vi "ABFL1dll.vi"(8 "error in (no error)":errorcluster, 11 "Inputs":T2) -> (0 "error out":errorcluster, 3 "Outputs":T1)   [LabVIEW 2015]
doc: "SINGLE-PHASE FLASH SUBROUTINES\n\nsubroutine ABFL1dll(a, b, z, kph, ab, dmin, dmax, t, p, D, ierr, herr, ab_length, herr_length)\n\nGeneral single-phase flash routine given two inputs and composition. \n\nValid input properties are temperature, pressure, density, energy, enthalpy, or entropy. \n\nThe character string ab specifies the inputs, which can be: T, P,D, E, H, S. An input of ‘EH’ (or ‘HE’) is not supported. The letters in this string must be uppercase.\n\nCare must be taken when sending inputs of T, P, or D, so that the same variable is not sent twice. For example,\nthe following would be wrong: call ABFL1 (‘TH’,T,H,z,kph,0,0,Dmin,Dmax,T,P,D,ierr,herr) \nRather, the following are examples of correct inputs: call ABFL1 (‘TH’,T,H,z,kph,0,0,Dmin,Dmax,tt,P, D,ierr,herr)\ncall ABFL1 (‘TP’,T,P,z,kph,0,0,Dmin,Dmax,tt,pp,D,ierr,herr) call ABFL1 (‘DS’,D,S,z,kph,0,0,Dmin,Dmax,T, P,dd,ierr,herr)\n\nThis routine accepts only single-phase inputs, it is intended primarily for use with the more general flash routine\nABFLSH, but can be called independently for increased calculation speed if the inputs are know to be singlephase.\nThis will avoid the call to the flash routines to determine the phase of the inputs. If this routine is called,\nbut the inputs are 2-phase, either an incorrect root or a metastable state will be returned (which is OK if the\nmetastable state is desired).\n\nINPUTS:\na -- First property (either temperature, pressure, density, entropy)\nb -- Second property (pressure, density, energy, enthalpy, or entropy)\nz -- Composition (array of mole fractions)\nkph -- Phase flag: 1 - Liquid (kph is only needed for TP inputs) 2 - Vapor\nab -- Character*2 string defining the inputs, e.g., ‘TH’ or ‘PS’ Valid characters\n are: T, P, D, E, H, S\ndmin -- Lower bound on density [mol/L] (for T inputs)\ndmax -- Upper bound on density [mol/L] (for T inputs)\n\nOUTPUTS:\nt -- Temperature [K]\np -- Pressure [kPa]\nD -- Molar density [mol/L]\nierr -- Error flag: 0 Successful, 248 Single-phase iteration did not converge\nherr -- Error string (character*255 variable if ierr<>0)\nab_length -- length of variable ab (default: 2)\nherr_length -- length of variable herr (default: 255) Flags ierr flags"
uses:
  REFPROP.dll
panel:
  # "REFPROP-ABFL1dll.vi"
  # "void  ABFL1dll(double *a, double *b, double *z, int32_t *kph, CStr ab, double *dmin, double *dmax, double *t, double *p, double *D, int32_t *ierr, CStr herr, int32_t ab_length, int32_t herr_length)"
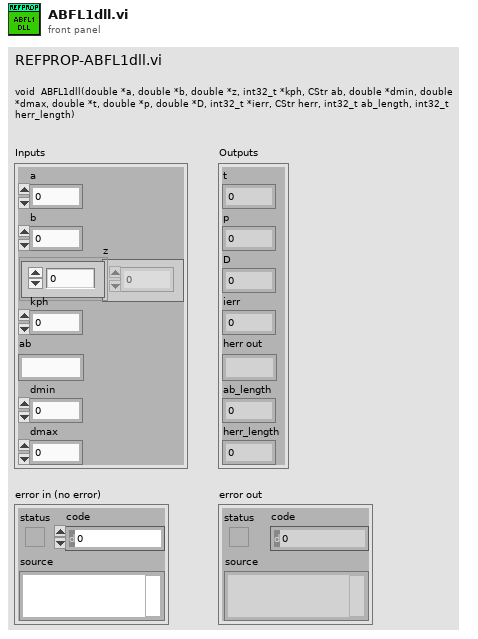
[diagram p1: front panel]
types:
  T1 = cluster{"t":dbl, "p":dbl, "D":dbl, "ierr":i32, "herr out":string, "ab_length":i32, "herr_length":i32}
  T2 = cluster{"a":dbl, "b":dbl, "z":dbl[], "kph":i32, "ab":string, "dmin":dbl, "dmax":dbl}
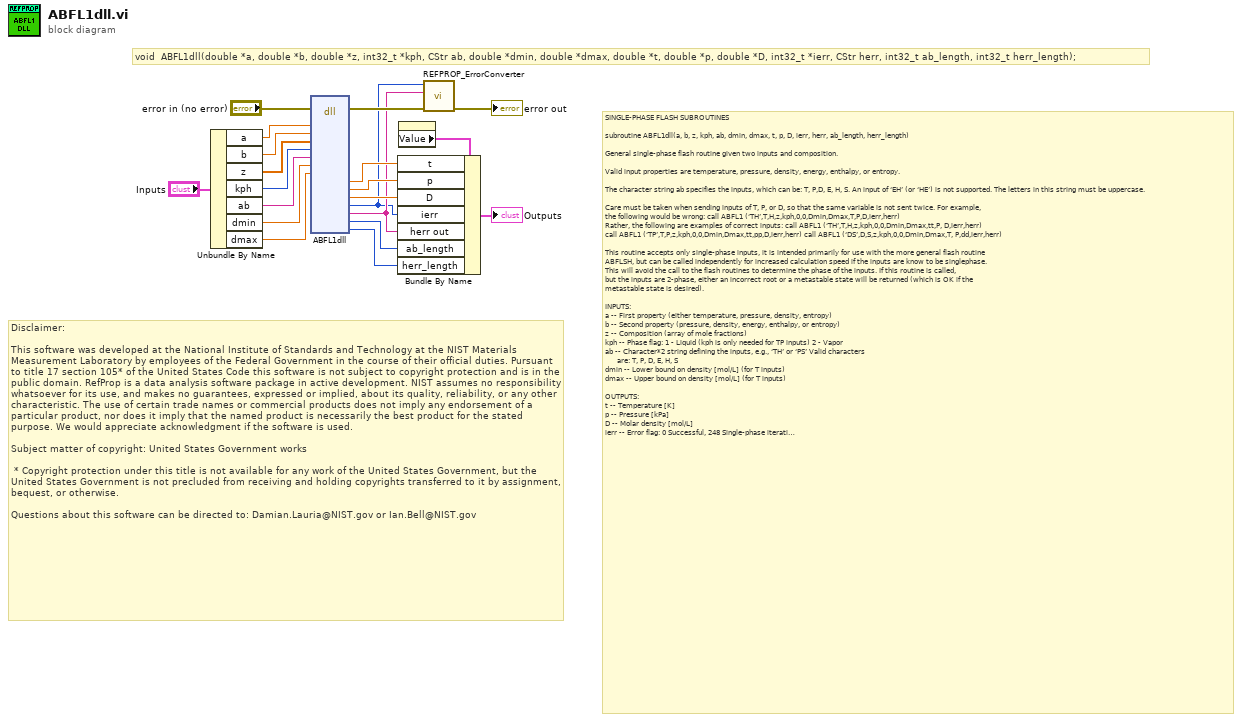
[diagram p0: block diagram]
diagram:
  # "Disclaimer:\n\nThis software was developed at the National Institute of Standards and Technology at the NIST Materials Measurement Laboratory by employees of the Federal Government in the course of their official duties. Pursuant to title 17 section 105* of the United States Code this software is not subject to copyright protection and is in the public domain. RefProp is a data analysis software package in active development. NIST assumes no responsibility whatsoever for its use, and makes no guarantees, expressed or implied, about its quality, reliability, or any other characteristic. The use of certain trade names or commercial products does not imply any endorsement of a particular product, nor does it imply that the named product is necessarily the best product for the stated purpose. We would appreciate acknowledgment if the software is used.\n \nSubject matter of copyright: United States Government works\n  \n * Copyright protection under this title is not available for any work of the United States Government, but the United States Government is not precluded from receiving and holding copyrights transferred to it by assignment, bequest, or otherwise.\n\nQuestions about this software can be directed to: Damian.Lauria@NIST.gov or Ian.Bell@NIST.gov"
  # "void  ABFL1dll(double *a, double *b, double *z, int32_t *kph, CStr ab, double *dmin, double *dmax, double *t, double *p, double *D, int32_t *ierr, CStr herr, int32_t ab_length, int32_t herr_length);"
  # "SINGLE-PHASE FLASH SUBROUTINES\n\nsubroutine ABFL1dll(a, b, z, kph, ab, dmin, dmax, t, p, D, ierr, herr, ab_length, herr_length)\n\nGeneral single-phase flash routine given two inputs and composition. \n\nValid input properties are temperature, pressure, density, energy, enthalpy, or entropy. \n\nThe character string ab specifies the inputs, which can be: T, P,D, E, H, S. An input of ‘EH’ (or ‘HE’) is not supported. The letters in this string must be uppercase.\n\nCare must be taken when sending inputs of T, P, or D, so that the same variable is not sent twice. For example,\nthe following would be wrong: call ABFL1 (‘TH’,T,H,z,kph,0,0,Dmin,Dmax,T,P,D,ierr,herr) \nRather, the following are examples of correct inputs: call ABFL1 (‘TH’,T,H,z,kph,0,0,Dmin,Dmax,tt,P, D,ierr,herr)\ncall ABFL1 (‘TP’,T,P,z,kph,0,0,Dmin,Dmax,tt,pp,D,ierr,herr) call ABFL1 (‘DS’,D,S,z,kph,0,0,Dmin,Dmax,T, P,dd,ierr,herr)\n\nThis routine accepts only single-phase inputs, it is intended primarily for use with the more general flash routine\nABFLSH, but can be called independently for increased calculation speed if the inputs are know to be singlephase.\nThis will avoid the call to the flash routines to determine the phase of the inputs. If this routine is called,\nbut the inputs are 2-phase, either an incorrect root or a metastable state will be returned (which is OK if the\nmetastable state is desired).\n\nINPUTS:\na -- First property (either temperature, pressure, density, entropy)\nb -- Second property (pressure, density, energy, enthalpy, or entropy)\nz -- Composition (array of mole fractions)\nkph -- Phase flag: 1 - Liquid (kph is only needed for TP inputs) 2 - Vapor\nab -- Character*2 string defining the inputs, e.g., ‘TH’ or ‘PS’ Valid characters\n      are: T, P, D, E, H, S\ndmin -- Lower bound on density [mol/L] (for T inputs)\ndmax -- Upper bound on density [mol/L] (for T inputs)\n\nOUTPUTS:\nt -- Temperature [K]\np -- Pressure [kPa]\nD -- Molar density [mol/L]\nierr -- Error flag: 0 Successful, 248 Single-phase iteration did not converge\nherr -- Error string (character*255 variable if ierr<>0)\nab_length -- length of variable ab (default: 2)\nherr_length -- length of variable herr (default: 255) Flags ierr flags"
  n1 = Unbundle By Name("Inputs") -> ("a"=w14:dbl, "b"=w13:dbl, "z"=w12:dbl[], "kph"=w11:i32, "ab"=w10:string, "dmin"=w9:dbl, "dmax"=w8:dbl)
  n2 = dll-call lib="C:/Users/lauria/Desktop/REFPROP 10 LabVIEW Wrapper BETA/REFPROP/REFPROP.*" fn="ABFL1dll"(error in="error in (no error)", "a"=w14, "b"=w13, "z"=w12, "kph"=w11, "ab"=w10, "dmin"=w9, "dmax"=w8) -> (error out=w20:errorcluster, "t"=w7:dbl, "p"=w6:dbl, "D"=w5:dbl, "ierr"=w1:i32, "herr"=w2:string, "ab_length"=w4:i32, "herr_length"=w3:i32)  [unwired: 17 in, 1 out]
  n3 = property on="Outputs" class="Clust (strict)"() -> ("Value"=w15:T1)  [unwired: 2 in, 2 out]
  n4 = Bundle By Name(cluster=w15, "t"=w7, "p"=w6, "D"=w5, "ierr"=w1, "herr out"=w2, "ab_length"=w4, "herr_length"=w3) -> (→"Outputs":T1)
  n5 = call "REFPROP_ErrorConverter.vi"("error in (no error)"=w20, "Error Message"=w2, "Error Code"=w1) -> ("error out"=→"error out":errorcluster)  [unwired: 8 in]
